vi "Update Message.vi"(8 "error in (no error)":errorcluster, 10 "Message":string, 11 "Chat Room Model in":refnum<class "Chat Room Model.lvclass">) -> (0 "error out":errorcluster, 3 "Chat Room Model out":refnum<class "Chat Room Model.lvclass">)   [LabVIEW 2025, in "Chat Room Model.lvlib" / "Chat Room Model.lvclass"]
uses:
  Chat Room Model.lvclass
  Chat Room Model.lvclass/Chat Room Model.ctl
  Chat Room Controller/Chat Room Controller Messages/Update Message Msg/Update Message Msg.lvclass
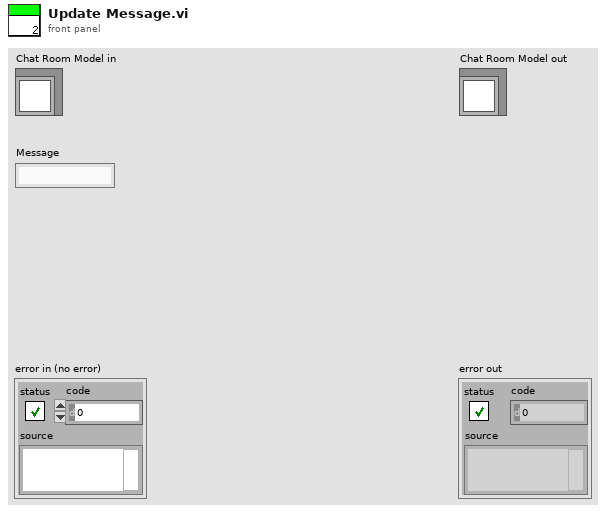
[diagram p1: front panel]
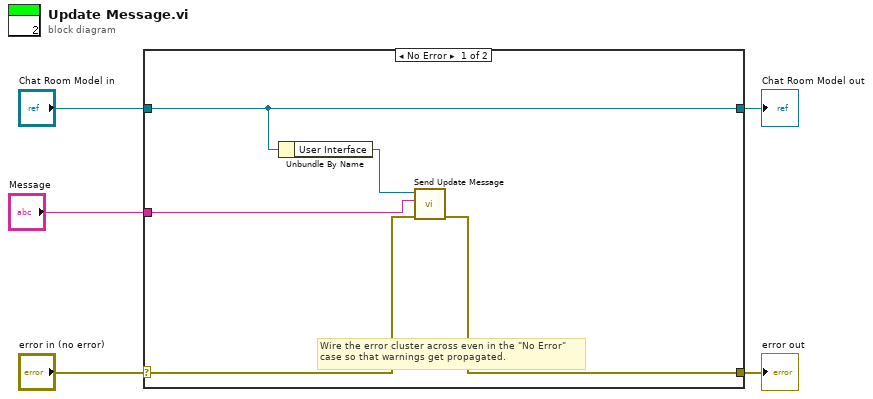
[diagram p0: block diagram]
diagram:
  n1 = case shown="No Error" "error in (no error)" {
    selector: "error in (no error)" -> [w7 w12]
    tunnel: [w6 w12] -> w4
    tunnel: [w10 w11] -> w2
    tunnel: "Chat Room Model in" -> [w10 w11]
    tunnel: "Message" -> [w8 _]
    frame No Error {
      # "Wire the error cluster across even in the \"No Error\"\ncase so that warnings get propagated."
      n2 = Unbundle By Name(w10) -> ("User Interface"=w9:refnum<class "Message Enqueuer.lvclass">)
      n3 = call "Send Update Message.vi"("error in (no error)"=w7, "Message"=w8, "Message Enqueuer"=w9) -> ("error out"=w6:errorcluster)  [unwired: 7 in, 1 out]
    }
    frame Error {
    }
  }
  "error out" <- w4
  "Chat Room Model out" <- w2
